vi "Set Attribute U32.vi"(8 "error in":errorcluster, 9 "Value":u32, 10 "Attribute":string, 11 "Config from JSON in":refnum<class "Config from JSON.lvclass">) -> (0 "error out":errorcluster, 3 "Config from JSON out":refnum<class "Config from JSON.lvclass">)   [LabVIEW 2025, in "Config from JSON.lvclass"]
uses:
  Config from JSON.lvclass
  Config from JSON.lvclass/Config from JSON.ctl
  e8263bad-b3ba-4f6f-aece-ecb16060d883.vi
  <vilib>/JDP Science/JSONtext/Variant to JSON Text.vi
  <vilib>/JDP Science/JSONtext/Set Item.vi
  <vilib>/JDP Science/JSONtext/LVClass Serializer/JSONtext LVClass Serializer.lvclass
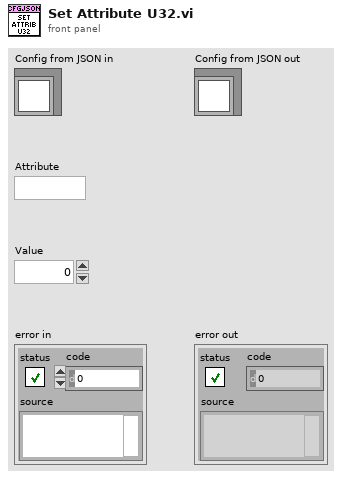
[diagram p1: front panel]
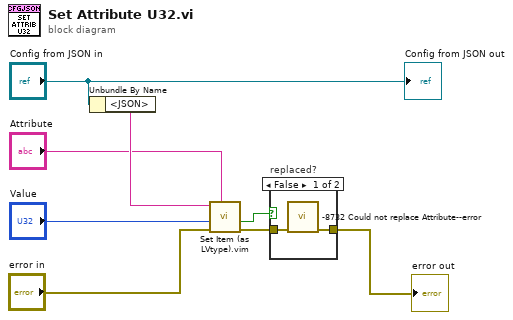
[diagram p0: block diagram]
diagram:
  n1 = Unbundle By Name("Config from JSON in") -> ("<JSON>"=w7:string)
  n2 = call "Set Item (as LVtype).vim"("$Path or Item Name"="Attribute", "error in (no error)"="error in", "Anything"="Value", "JSON"=w7) -> ("error out"=w4:errorcluster, "Replaced"=w1:bool)  [unwired: 4 in, 1 out]
  n3 = case "replaced?" shown="False" w1 {
    tunnel: w4 -> [w10 w11]
    tunnel: [w9 w11] -> w2
    frame False {
      n4 = call "-8732 Could not replace Attribute--error.vi"("error in"=w10) -> ("error out"=w9:errorcluster)  [unwired: 10 in]
    }
    frame True {
    }
  }
  "error out" <- w2
  "Config from JSON out" <- "Config from JSON in"
